vi "Set SMU Voltage.vi"(8 "error in (no error)":errorcluster, 9 "VDD voltage level":dbl=1.8 caption="voltage level" format="%_6p", 10 "Pins":string[](array[string])=["VDD"], 11 "Semiconductor Module Context":T1) -> (0 "error out":errorcluster, 2 "Instrument Sessions Out":refnum<k15>[](array[refnum]), 3 "Semiconductor Module Context Out":T1)   [LabVIEW 2013]
uses:
  <vilib>/NI_TestStand_SemiconductorModule/NI_TestStand_Semiconductor_Module.lvlibp/PinMap/General/SemiconductorModuleContext.ctl
  <vilib>/NI_TestStand_SemiconductorModule/NI_TestStand_Semiconductor_Module.lvlibp/PinMap/DC Power/PinsToNIDCPowerSessions.vi
  <vilib>/NI_TestStand_SemiconductorModule/NI_TestStand_Semiconductor_Module.lvlibp
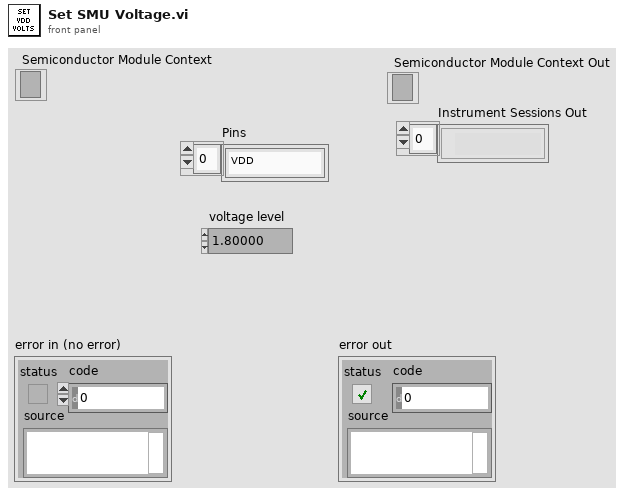
[diagram p1: front panel]
types:
  T1 = typedef "NI_TestStand_Semiconductor_Module.lvlibp/SemiconductorModuleContext.ctl" = refnum<k7>
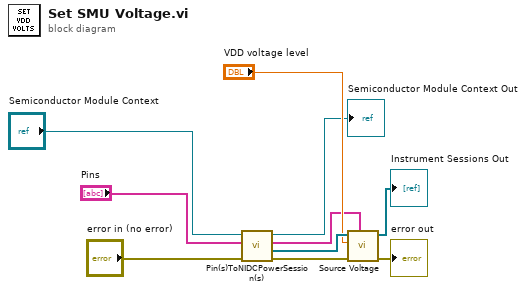
[diagram p0: block diagram]
diagram:
  n1 = call-poly <vilib>:"Pin(s)ToNIDCPowerSession(s).vi"("error in (no error)"="error in (no error)", "Pins"="Pins", "Semiconductor Module Context"="Semiconductor Module Context") -> ("error out"=w8:errorcluster, "Instrument Sessions"=w6:refnum<k15>[], "Channel Lists"=w4:string[], "Semiconductor Module Context Out"=→"Semiconductor Module Context Out":T1)  [unwired: 4 in, 1 out]
  n2 = call "Source Voltage.vi"("Channel Lists"=w4, "error in (no error)"=w8, "voltage level"="VDD voltage level", "Instrument Sessions In"=w6) -> ("error out"=→"error out":errorcluster, "Instrument Sessions Out"=→"Instrument Sessions Out":refnum<k15>[])  [unwired: 4 in, 2 out]
